vi "Update Chart Data.vi"(8 "error in (no error)":errorcluster, 9 "Limits":T1, 10 "Value":dbl, 11 "WaveformChart in":refnum<vi>) -> (0 "error out":errorcluster)   [LabVIEW 2014, in "Chart Module.lvlib"]
uses:
  Chart Module.lvlib
  Limits Argument--cluster.ctl
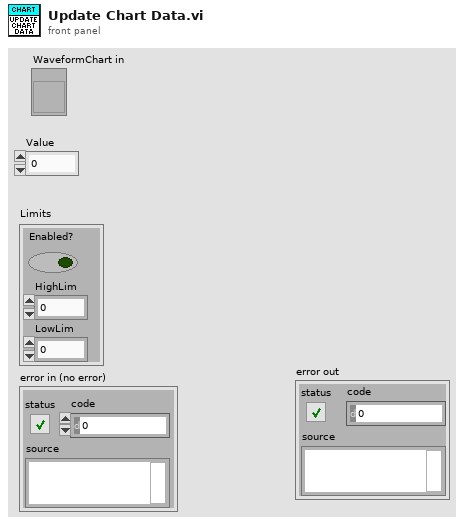
[diagram p1: front panel]
types:
  T1 = typedef "Chart Module.lvlib/Limits Argument--cluster.ctl" = cluster{"Enabled?":bool, "HighLim":dbl, "LowLim":dbl}
  T2 = cluster{"Value":dbl, "HighLim":dbl, "LowLim":dbl}
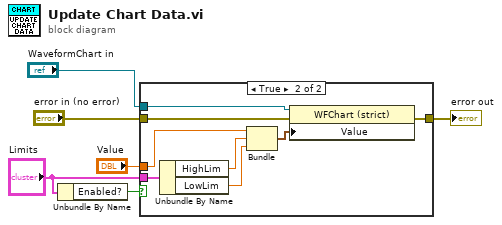
[diagram p0: block diagram]
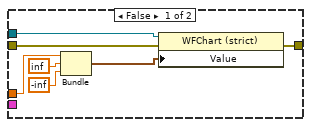
[diagram p2: hidden frame]
diagram:
  n1 = Unbundle By Name("Limits") -> ("Enabled?"=w2:bool)
  n2 = case shown="True" w2 {
    tunnel: "Value" -> [w13 w21]
    tunnel: "WaveformChart in" -> [w9 w19]
    tunnel: [w7 w18] -> w4
    tunnel: "error in (no error)" -> [w8 w17]
    tunnel: "Limits" -> [_ w16]
    frame False {
      n3 = Bundle("Value"=w13, "HighLim"=inf, "LowLim"=-inf) -> (w10:T2)  [unwired: 1 in]
      n4 = property class="WFChart (strict)"(reference=w9, error in=w8, "Value"=w10) -> (error out=w7:errorcluster)  [unwired: 1 out]
    }
    frame True {
      n5 = Unbundle By Name(w16) -> ("HighLim"=w15:dbl, "LowLim"=w14:dbl)
      n6 = Bundle("Value"=w21, "HighLim"=w15, "LowLim"=w14) -> (w20:T2)  [unwired: 1 in]
      n7 = property class="WFChart (strict)"(reference=w19, error in=w17, "Value"=w20) -> (error out=w18:errorcluster)  [unwired: 1 out]
    }
  }
  "error out" <- w4
